vi "StartServerVi.vi"(0 "Baxter":T2) -> (1 "Active Topics":T1(array[cluster]), 2 "Reply":string, 3 "Baxter out":T2)   [LabVIEW 2010]
uses:
  <userlib>/ROSforLV_0.1/ROS/Code/SubVIs/_ROSControl.ctl
  <userlib>/ROSforLV_0.1/ROS/Code/SubVIs/_ROSDirection.ctl
  <userlib>/ROSforLV_0.1/ROS/Code/_ROSDefinition.vi
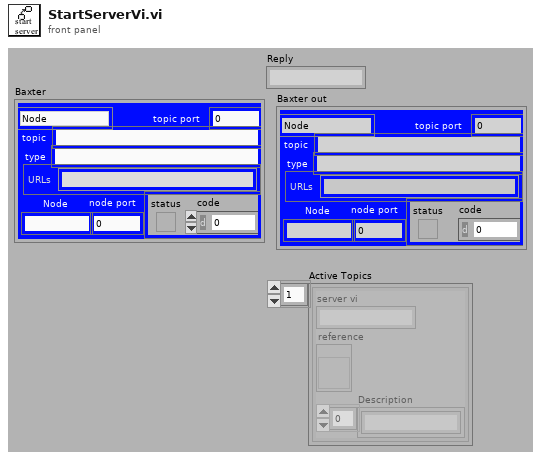
[diagram p1: front panel]
types:
  T1 = cluster{"server vi":string, "reference":refnum<vi>, "Description":string[]}[]
  T2 = typedef "_ROSControl.ctl" = cluster{"topic port":u16, "Node":string, "topic":string, "type":string, "node port":u32, "error ":errorcluster, "Direction":T3, "APIs":string[]}
  T3 = typedef "_ROSDirection.ctl" = enum16{"Node", "Publisher", "Subscriber", "Service Client"}
  T4 = enum32{"Bad", "Idle", "Run top level", "Running"}
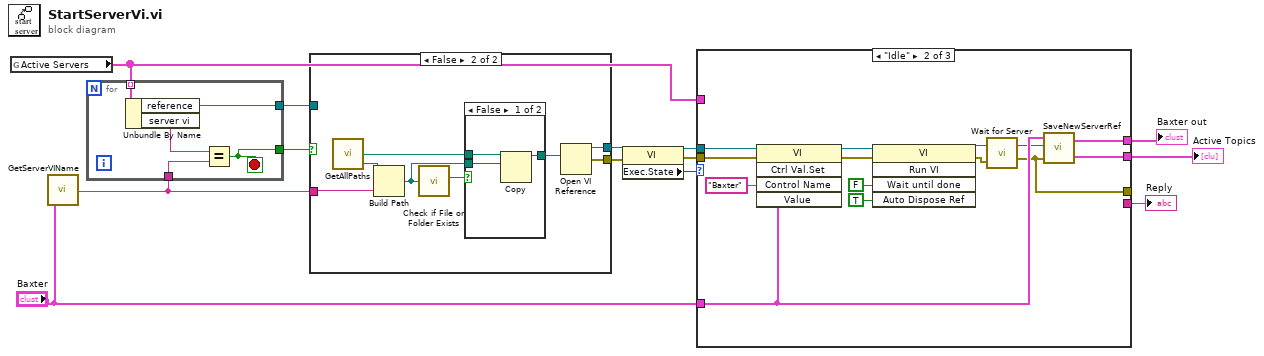
[diagram p0: block diagram]
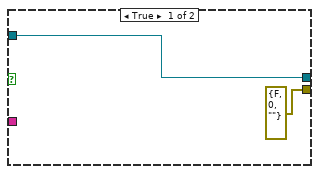
[diagram p2: hidden frame]
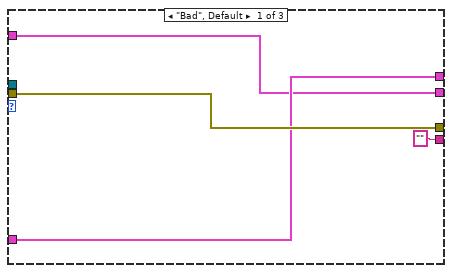
[diagram p4: hidden frame]
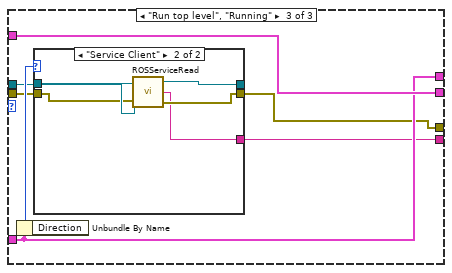
[diagram p5: hidden frame]
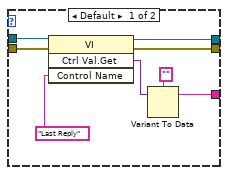
[diagram p6: hidden frame]
diagram:
  n1 = global read "_ROSDefinition.vi" "Active Servers"() -> (w1:T1)
  n2 = call <userlib>:"GetServerVIName.vi"("Baxter"="Baxter") -> ("vi name"=w5:string)
  n3 = for {
    tunnel: w1 -> [w18] mode=indexing
    tunnel: w5 -> [w16]
    tunnel: [w15] -> w4
    tunnel: [w14] -> w3
    stop <- w15 stop-if-true
    n4 = Unbundle By Name(w18) -> ("reference"=w14:refnum<vi>, "server vi"=w17:string)
    n5 = Equal?(x=w17, y=w16) -> (x = y?=w15:bool)
  }
  n6 = case shown="False" w4 {
    tunnel: w5 -> [_ w28]
    tunnel: [w19 w22] -> w12
    tunnel: [errorcluster {"status"=FALSE, "code"=0, "source"=""} ("error out") w21] -> w11
    tunnel: w3 -> [w19 _]
    frame True {
    }
    frame False {
      n7 = call <userlib>:"GetAllPaths.vi"() -> ("Server Folder"=w23:path, "BlankServer"=w24:path)  [unwired: 1 in, 1 out]
      n8 = Build Path(base path=w23, name or relative path=w28) -> (appended path=w26:path)
      n9 = call <vilib>:"Check if File or Folder Exists.vi"("path"=w26) -> ("file or folder exists?"=w25:bool)  [unwired: 8 in, 2 out]
      n10 = case shown="False" w25 {
        tunnel: w24 -> [w31 _]
        tunnel: w26 -> [w30 w32]
        tunnel: [w29 w32] -> w27
        frame False {
          n11 = Copy(10:w30, 11:w31) -> (3:w29:path)  [unwired: 3 in, 2 out]
        }
        frame True {
        }
      }
      n12 = Open VI Reference(vi path=w27) -> (vi reference=w22:refnum<vi>, error out=w21:errorcluster)  [unwired: 5 in]
    }
  }
  n13 = property class="VI"(reference=w12, error in=w11) -> (reference out=w9:refnum<vi>, error out=w8:errorcluster, "Exec.State"=w10:T4)
  n14 = case shown="\"Idle\"" w10 {
    tunnel: w9 -> [_ w48 w54]
    tunnel: [w36 w40 w52] -> _
    tunnel: w8 -> [w36 w45 w53]
    tunnel: "Baxter" -> [w34 w44 w56]
    tunnel: ["" ("Control Name") _ w51] -> w13
    tunnel: [w34 w43 w56] -> w6
    tunnel: [w33 w42 w57] -> w2
    tunnel: w1 -> [w33 _ w57]
    frame "Bad", Default {
    }
    frame "Idle" {
      n15 = invoke class="VI" method="Ctrl Val.Set"(reference=w48, error in=w45, "Control Name"="Baxter", "Value"=w44) -> (reference out=w47:refnum<vi>, error out=w37:errorcluster)  [unwired: 1 in, 3 out]
      n16 = invoke class="VI" method="Run VI"(reference=w47, error in=w37, "Wait until done"=FALSE ("Wait Until Done"), "Auto Dispose Ref"=TRUE ("Wait Until Done")) -> (reference out=w38:refnum<vi>, error out=w39:errorcluster)  [unwired: 1 in, 3 out]
      n17 = call "Wait for Server.vi"("error in"=w39, "vi reference in"=w38) -> ("error out"=w40:errorcluster, "vi reference out"=w41:refnum<vi>)
      n18 = call <userlib>:"SaveNewServerRef.vi"("error"=w40, "vi reference"=w41, "Baxter in"=w44) -> ("Active Topics"=w42:T1, "Baxter out"=w43:T2)
    }
    frame "Run top level", "Running" {
      n19 = Unbundle By Name(w56) -> ("Direction"=w55:T3)
      n20 = case shown="\"Service Client\"" w55 {
        tunnel: w54 -> [w62 w70]
        tunnel: w53 -> [w63 w67]
        tunnel: [w60 w69] -> _
        tunnel: [w61 w68] -> w52
        tunnel: [w58 w66] -> w51
        frame Default {
          n21 = invoke class="VI" method="Ctrl Val.Get"(reference=w62, error in=w63, "Control Name"="Last Reply") -> (reference out=w60:refnum<vi>, error out=w61:errorcluster, "Get Control Value Variant"=w64:variant)  [unwired: 1 in, 1 out]
          n22 = Variant To Data(Variant=w64, type="" ("Control Name")) -> (data=w58:string)  [unwired: 1 in, 1 out]
        }
        frame "Service Client" {
          n23 = call <userlib>:"ROSServiceRead.vi"("error in"=w67, "vi reference"=w70) -> ("error out"=w68:errorcluster, "Reply"=w66:string, "vi reference"=w69:refnum<vi>)
        }
      }
    }
  }
  "Baxter out" <- w6
  "Reply" <- w13
  "Active Topics" <- w2
